vi "Mode Scan Engine.vi"() -> ()   [LabVIEW 2014]
uses:
  Controls/Standard Action.ctl
  DM_Single_V2/Controls/Standard_Counter_Action.ctl
  <vilib>/Analysis/6fits.llb/Curve Fitting Criteria.ctl
  <vilib>/Analysis/baseanly.llb/Mean (DBL).vi
  <vilib>/Analysis/NI_AALBase.lvlib
  <vilib>/Analysis/NI_AALPro.lvlib
  <vilib>/gmath/NI_Gmath.lvlib
panel:
  in  "Initial Guess":T1={"Amp"=25.0, "Center"=0.0, "Sigma"=1.0, "Offset"=0.0}
  in  "Manual Initial Guess":bool=TRUE
  in  "Upper Limit":dbl=100.0
  in  "Lower Limit":dbl=20.0
  out "Metric":cluster{dbl[], dbl[]}[](graph)
  out "Image":sgl[][](graph)
  in  "Step Size":dbl=0.5
  in  "Number of Steps":u16=9
  in  "Get Image":bool
  in  "Scan Next Mode":bool
  in  "Metric":u16(ring) items=["Max Intensity", "No Zero Mean", "Threshold Mean"]
  in  "Fit Type":u16(ring) items=["Guassian", "Quadratic"]
  in  "Mode":i32(ring) items=["1", "1"]
  in  "Apply":bool
  in  "Fit Data":bool
  in  "Scan Mode":bool
  in  "Exit":bool
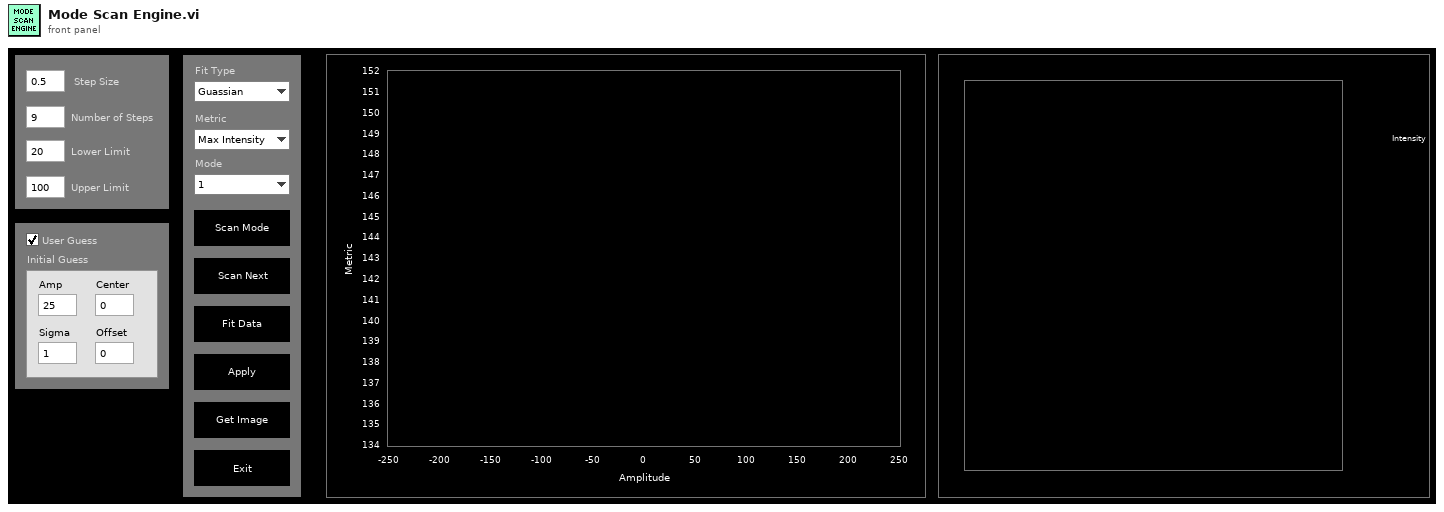
[diagram p1: front panel]
types:
  T1 = cluster{"Amp":dbl, "Center":dbl, "Sigma":dbl, "Offset":dbl}
  T2 = typedef "Standard Action.ctl" = enum16{"Read", "Write"}
  T3 = typedef "MirrorModes_DUAL.ctl" = cluster{"Mode":string, "Amplitude":dbl}[][]
  T4 = typedef "Standard_Counter_Action.ctl" = enum16{"Initialize", "Update Count", "Get Count"}
  T5 = cluster{"amp min":dbl, "amp max":dbl, "center min":dbl, "center max":dbl, "deviation min":dbl, "deviation max":dbl, "offset min":dbl, "offset max":dbl}
  T6 = enum16{"Linear", "Polynomial", "Exponential", "Power"}
  T7 = cluster{"Amplitude Out":dbl[], "Metric Out":dbl[]}
  T8 = cluster{"Amp":dbl, "Numeric":dbl, "Sigma":dbl, "Offset":dbl}
  T9 = typedef "NI_AALPro.lvlib/Curve Fitting Criteria.ctl" = u16
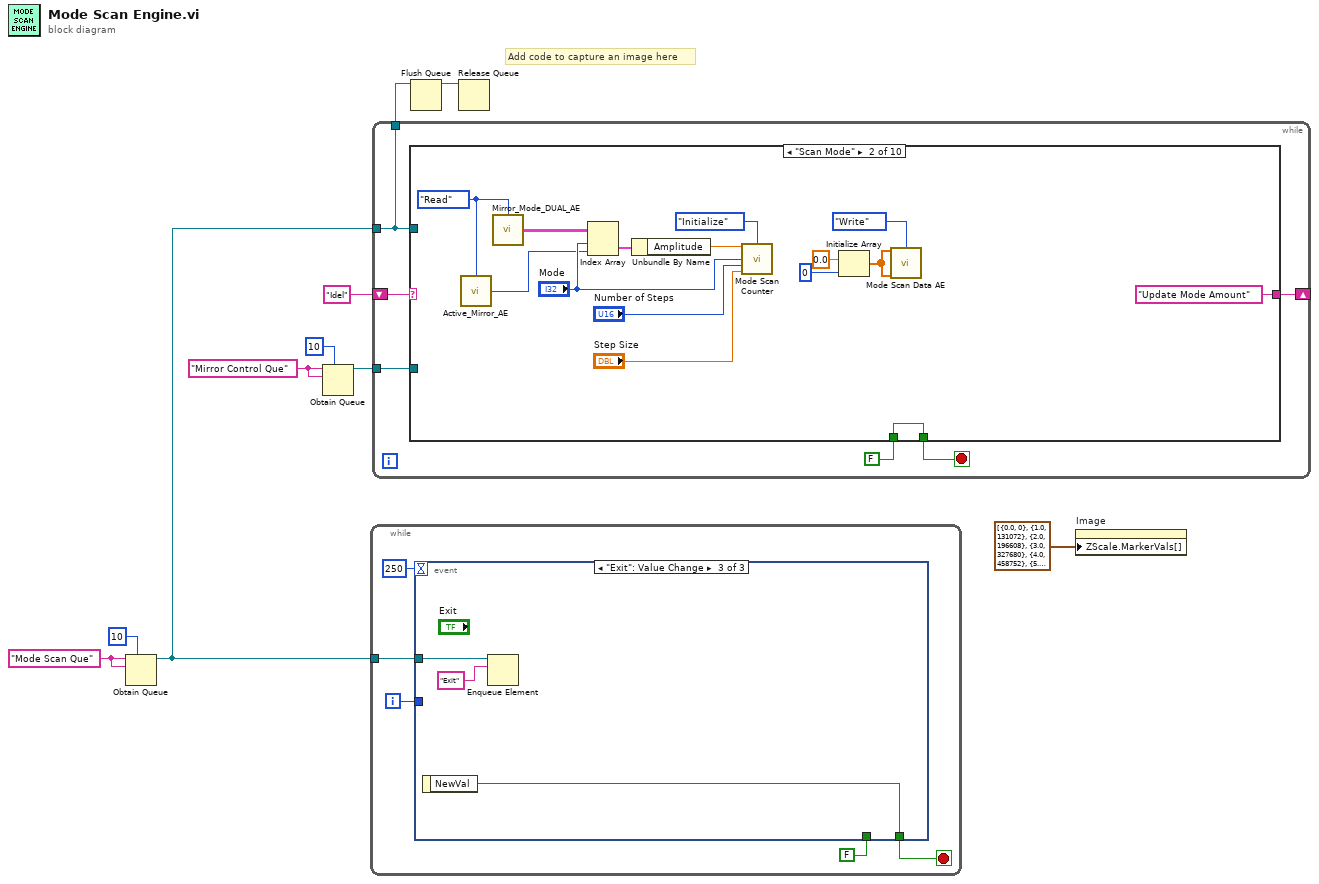
[diagram p0: block diagram]
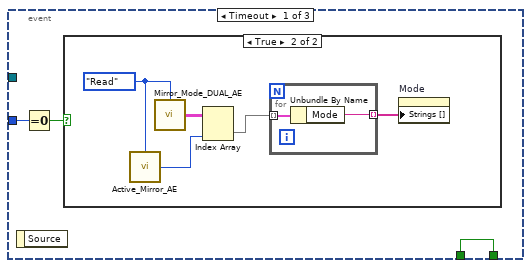
[diagram p2: hidden frame]
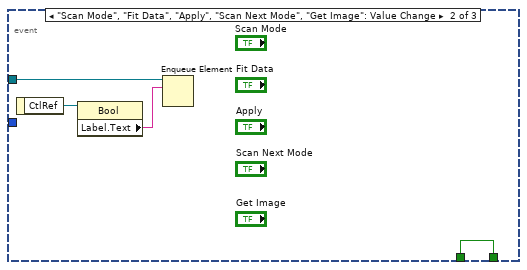
[diagram p4: hidden frame]
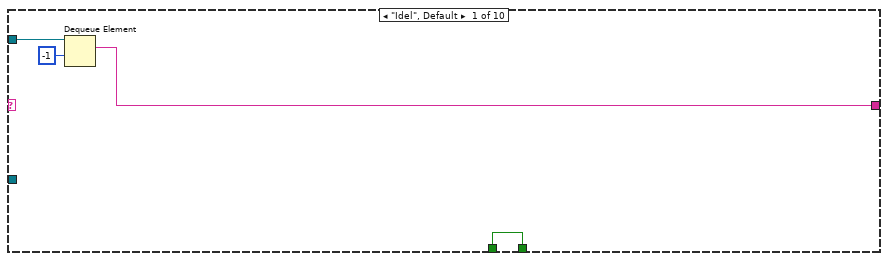
[diagram p5: hidden frame]
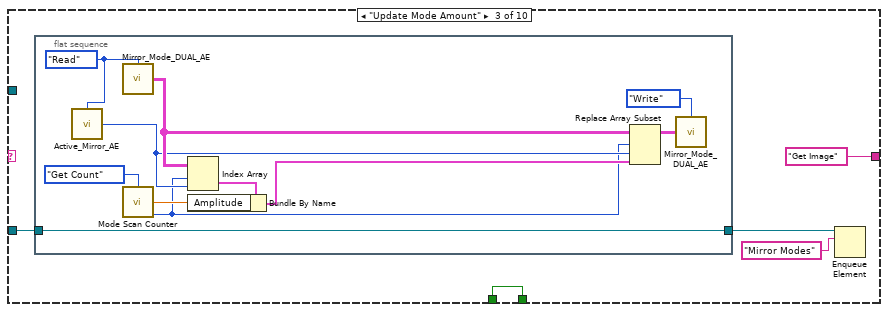
[diagram p6: hidden frame]
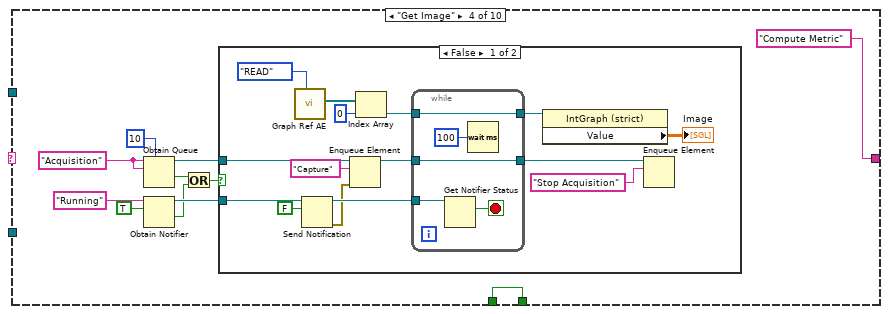
[diagram p7: hidden frame]
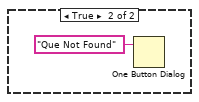
[diagram p8: hidden frame]
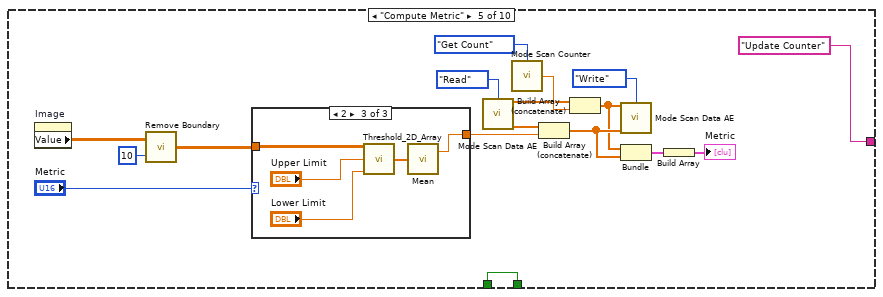
[diagram p9: hidden frame]
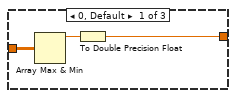
[diagram p10: hidden frame]
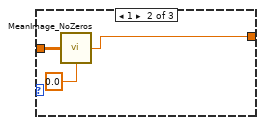
[diagram p11: hidden frame]
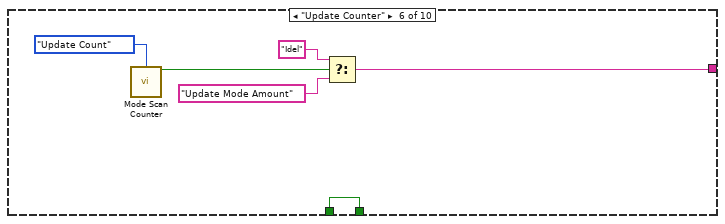
[diagram p12: hidden frame]
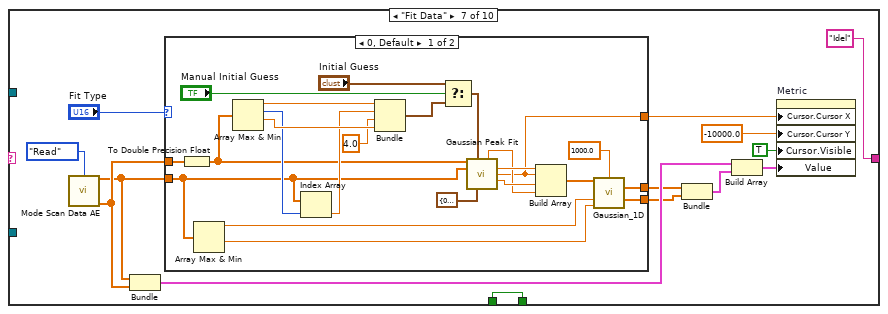
[diagram p13: hidden frame]
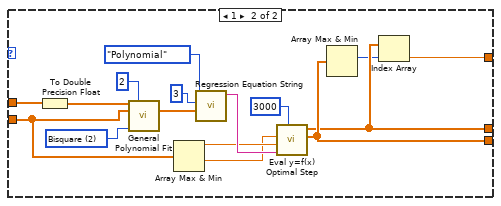
[diagram p14: hidden frame]
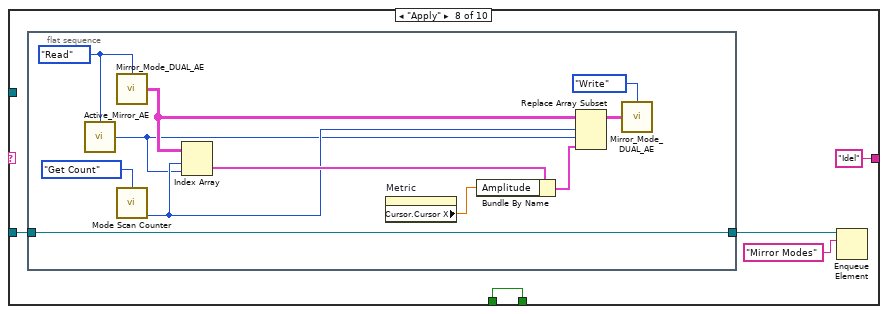
[diagram p15: hidden frame]
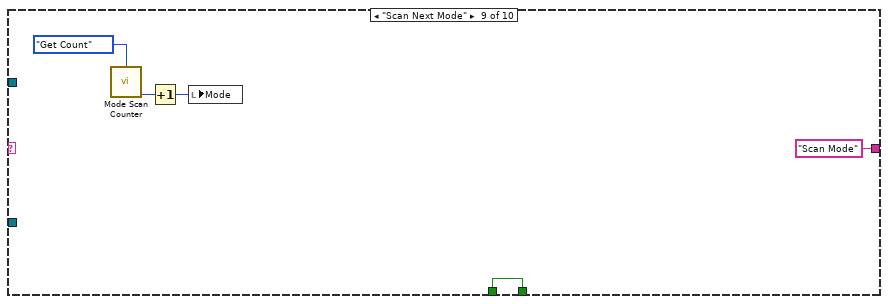
[diagram p16: hidden frame]
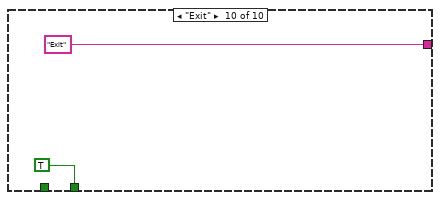
[diagram p17: hidden frame]
diagram:
  w4 = "Mirror Control Que" ("name (unnamed)")
  w9 = "Mode Scan Que" ("name (unnamed)")
  # "Add code to capture an image here"
  n1 = Obtain Queue(max queue size (-1, unlimited)=10, name (unnamed)=w9, element data type=w9) -> (queue out=w7:refnum<queue>)  [unwired: 2 in, 2 out]
  n2 = Obtain Queue(max queue size (-1, unlimited)=10, name (unnamed)=w4, element data type=w4) -> (queue out=w2:refnum<queue>)  [unwired: 2 in, 2 out]
  n3 = while {
    tunnel: w7 -> [w15]
    i -> [w12]
    stop <- w14 stop-if-true
    n4 = event shown="[2] \"Exit\": Value Change" {
      selector: _ -> [_ _ _]
      dyn-events: _ -> [_ _ _]
      timeout: 250 -> [_ _ _]
      tunnel: w15 -> [_ w28 w32]
      tunnel: [w18 w26 w30] -> w14
      tunnel: FALSE -> [w18 w26 _]
      tunnel: w12 -> [w17 _ _]
      event Timeout {
        n5 = event-data() -> ()  [unwired: 1 in, 1 out]
        n6 = Equal To 0?(x=w17) -> (x = 0?=w16:bool)
        n7 = case shown="True" w16 {
          frame False {
          }
          frame True {
            w22 = Standard_Action."Read" ("Action")
            n8 = call "Active_Mirror_AE.vi"("Action"=w22) -> ("Active Mirror"=w19:i32)  [unwired: 14 in]
            n9 = call "Mirror_Mode_DUAL_AE.vi"("Action"=w22) -> ("Mirror Modes Out"=w21:T3)  [unwired: 14 in]
            n10 = Index Array(array=w21, index (col)=w19) -> (element=w20:cluster{"Mode":string, "Amplitude":dbl}[])  [unwired: 1 in]
            n11 = for {
              tunnel: w20 -> [w25] mode=indexing
              tunnel: [w24] -> w23 mode=indexing
              n12 = Unbundle By Name(w25) -> ("Mode"=w24:string)
            }
            n13 = property on="Mode" class="Ring (strict)"("Strings []"=w23) -> ()  [unwired: 2 in, 2 out]
          }
        }
      }
      event "Scan Mode", "Fit Data", "Apply", "Scan Next Mode", "Get Image": Value Change {
        n14 = event-data() -> ("CtlRef"=w27:refnum<vi>)  [unwired: 1 in]
        n15 = property class="Bool"(reference=w27) -> ("Label.Text"=w29:string)  [unwired: 1 in, 2 out]
        n16 = Enqueue Element(queue=w28, element=w29) -> ()  [unwired: 2 in, 3 out]
      }
      event "Exit": Value Change {
        n17 = event-data() -> ("NewVal"=w30:bool)  [unwired: 1 in]
        n18 = Enqueue Element(queue=w32, element="Exit") -> ()  [unwired: 2 in, 3 out]
      }
    }
  }
  n19 = while {
    shift-right: [w35] -> _
    shift-left: "Idel" -> [w38]
    tunnel: w7 -> [w34]
    tunnel: [w34] -> w6
    tunnel: w2 -> [w33]
    stop <- w37 stop-if-true
    n20 = case shown="\"Scan Mode\"" w38 {
      tunnel: [w42 w57 w62 w84 w121 w139 w153 w197 w213 TRUE] -> w37
      tunnel: FALSE -> [w42 w57 w62 w84 w121 w139 w153 w197 w213 _]
      tunnel: w34 -> [w40 _ _ _ _ _ _ _ _ _]
      tunnel: [w39 "Update Mode Amount" ("name (unnamed)") "Get Image" ("name (unnamed)") "Compute Metric" ("name (unnamed)") "Update Counter" ("name (unnamed)") w136 "Idel" ("name (unnamed)") "Idel" ("name (unnamed)") "Scan Mode" ("name (unnamed)") "Exit" ("name (unnamed)")] -> w35
      tunnel: w33 -> [_ _ w61 _ _ _ _ w195 _ _]
      frame "Idel", Default {
        n21 = Dequeue Element(queue=w40, timeout in ms (-1)=-1) -> (element=w39:string)  [unwired: 1 in, 3 out]
      }
      frame "Scan Mode" {
        w45 = Standard_Action."Read" ("Action")
        n22 = call "Active_Mirror_AE.vi"("Action"=w45) -> ("Active Mirror"=w43:i32)  [unwired: 14 in]
        n23 = call "Mirror_Mode_DUAL_AE.vi"("Action"=w45) -> ("Mirror Modes Out"=w52:T3)  [unwired: 14 in]
        n24 = Index Array(array=w52, index (row)="Mode", index (col)=w43) -> (element=w53:cluster{"Mode":string, "Amplitude":dbl})
        n25 = Unbundle By Name(w53) -> ("Amplitude"=w54:dbl)
        n26 = call "Mode Scan Counter.vi"("Center Value"=w54, "Action"=Standard_Counter_Action."Initialize", "Mode"="Mode", "Number of Steps"="Number of Steps", "Step Size"="Step Size") -> ()  [unwired: 8 in, 3 out]
        n27 = Initialize Array(0.0 ("element"), 0 ("dimension size")) -> (w46:dbl[])
        n28 = call "Mode Scan Data AE.vi"("Amplitude"=w46, "Action"=Standard_Action."Write", "Metric"=w46) -> ()  [unwired: 11 in, 2 out]
      }
      frame "Update Mode Amount" {
        n29 = flat-sequence {
          tunnel: w61 -> [w66]
          tunnel: [w66] -> w59
          frame #0 {
            w65 = Standard_Action."Read" ("Action")
            n30 = call "Active_Mirror_AE.vi"("Action"=w65) -> ("Active Mirror"=w64:i32)  [unwired: 14 in]
            n31 = call "Mirror_Mode_DUAL_AE.vi"("Action"=w65) -> ("Mirror Modes Out"=w68:T3)  [unwired: 14 in]
            n32 = call "Mode Scan Counter.vi"("Action"=Standard_Counter_Action."Get Count") -> ("Output"=w72:dbl, "Current Mode"=w63:i32)  [unwired: 12 in, 1 out]
            n33 = Index Array(array=w68, index (row)=w63, index (col)=w64) -> (element=w71:cluster{"Mode":string, "Amplitude":dbl})
            n34 = Bundle By Name(cluster=w71, "Amplitude"=w72) -> (w73:cluster{"Mode":string, "Amplitude":dbl})
            n35 = Replace Array Subset(array=w68, new element=w73, index (row)=w63, index (col)=w64) -> (w70:T3)
            n36 = call "Mirror_Mode_DUAL_AE.vi"("Action"=Standard_Action."Write", "Mirror Modes In"=w70) -> ()  [unwired: 13 in, 1 out]
          }
        }
        n37 = Enqueue Element(queue=w59, element="Mirror Modes" ("name (unnamed)")) -> ()  [unwired: 2 in, 3 out]
      }
      frame "Get Image" {
        w79 = "Acquisition" ("name (unnamed)")
        n38 = Obtain Queue(max queue size (-1, unlimited)=10, name (unnamed)=w79, element data type=w79) -> (queue out=w82:refnum<queue>, created new?=w76:bool)  [unwired: 2 in, 1 out]
        n39 = Obtain Notifier(name (unnamed)="Running", notification data type=TRUE) -> (notifier out=w81:refnum<notifier>, created new?=w75:bool)  [unwired: 2 in, 1 out]
        n40 = Or(x=w76, y=w75) -> (x .or. y?=w74:bool)
        n41 = case shown="False" w74 {
          tunnel: w82 -> [w88 _]
          tunnel: w81 -> [w86 _]
          frame False {
            n42 = call "Graph Ref AE.vi"("Action"=enum16{"READ", "WRITE"}."READ") -> ("Graph Ref Out"=w96:refnum<vi>[])  [unwired: 10 in]
            n43 = Send Notification(notification=FALSE, notifier=w86) -> (notifier out=w91:refnum<notifier>, error out=w90:errorcluster)  [unwired: 1 in]
            n44 = Enqueue Element(queue=w88, element="Capture", error in (no error)=w90) -> (queue out=w92:refnum<queue>)  [unwired: 1 in, 2 out]
            n45 = Index Array(array=w96, index=0) -> (element=w98:refnum<vi>)
            n46 = while {
              tunnel: w91 -> [w104]
              tunnel: [w102] -> w93
              tunnel: w92 -> [w102]
              tunnel: [w101] -> w99
              tunnel: w98 -> [w101]
              stop <- w103 stop-if-true
              n47 = Get Notifier Status(notifier=w104) -> (current notification=w103:bool)  [unwired: 1 in, 4 out]
              n48 = Wait (ms)(milliseconds to wait=u32 100) -> ()  [unwired: 1 out]
            }
            n49 = property class="IntGraph (strict)"(reference=w99) -> ("Value"=→"Image":sgl[][])  [unwired: 1 in, 2 out]
            n50 = Enqueue Element(queue=w93, element="Stop Acquisition" ("f")) -> ()  [unwired: 2 in, 3 out]
          }
          frame True {
            n51 = One Button Dialog(message="Que Not Found") -> ()  [unwired: 1 in, 1 out]
          }
        }
      }
      frame "Compute Metric" {
        n52 = property on="Image" class="IntGraph (strict)"() -> ("Value"=w108:sgl[][])  [unwired: 2 in, 2 out]
        n53 = call "Remove Boundary.vi"("deleted pixel number"=10, "input"=w108) -> ("output"=w107:dbl[][])
        n54 = case shown="2" "Metric" {
          tunnel: w107 -> [w125 w128 w133]
          tunnel: [w123 w127 w131] -> w115
          frame 0, Default {
            n55 = Array Max & Min(array=w125) -> (max value=w124:dbl)  [unwired: 3 out]
            n56 = To Double Precision Float(number=w124) -> (double precision float=w123:dbl)
          }
          frame 1 {
            n57 = call "MeanImage_NoZeros.vi"("Image IN"=w128, "STDev Factor"=0.0) -> ("No Zero Mean"=w127:dbl)  [unwired: 13 in]
          }
          frame 2 {
            n58 = call "Threshold_2D_Array.vi"("2D Array IN"=w133, "Upper Limit"="Upper Limit", "Lower Limit"="Lower Limit") -> ("Threshold Array Out"=w132:dbl[])  [unwired: 12 in]
            n59 = call-poly <vilib>:"Mean.vi"("X"=w132) -> ("mean"=w131:dbl)  [unwired: 1 out]
          }
        }
        n60 = call "Mode Scan Data AE.vi"("Action"=Standard_Action."Read") -> ("Amplitude Out"=w112:dbl[], "Metric Out"=w113:dbl[])  [unwired: 13 in]
        n61 = call "Mode Scan Counter.vi"("Action"=Standard_Counter_Action."Get Count") -> ("Output"=w114:dbl)  [unwired: 12 in, 2 out]
        n62 = Build Array (concatenate)(w113, w115) -> (w118:dbl[])
        n63 = Build Array (concatenate)(w112, w114) -> (w117:dbl[])
        n64 = call "Mode Scan Data AE.vi"("Amplitude"=w117, "Action"=Standard_Action."Write", "Metric"=w118) -> ()  [unwired: 11 in, 2 out]
        n65 = Bundle(w117, w118) -> (w119:cluster{dbl[], dbl[]})  [unwired: 1 in]
        n66 = Build Array(w119) -> (→"Metric":cluster{dbl[], dbl[]}[])
      }
      frame "Update Counter" {
        n67 = call "Mode Scan Counter.vi"("Action"=Standard_Counter_Action."Update Count") -> ("Scan Done?"=w134:bool)  [unwired: 12 in, 2 out]
        n68 = Select(t="Idel", s=w134, f="Update Mode Amount") -> (s? t:f=w136:string)
      }
      frame "Fit Data" {
        n69 = call "Mode Scan Data AE.vi"("Action"=Standard_Action."Read") -> ("Amplitude Out"=w148:dbl[], "Metric Out"=w149:dbl[])  [unwired: 13 in]
        n70 = Bundle("Amplitude Out"=w148, "Metric Out"=w149) -> (w147:T7)  [unwired: 1 in]
        n71 = case shown="0, Default" "Fit Type" {
          tunnel: w148 -> [w169 w182]
          tunnel: w149 -> [w176 w181]
          tunnel: [w157 w178] -> w142
          tunnel: [w156 w179] -> w145
          tunnel: [w155 w180] -> w144
          frame 0, Default {
            n72 = To Double Precision Float(number=w176) -> (double precision float=w170:dbl[])
            n73 = Array Max & Min(array=w169) -> (max value=w158:dbl, min value=w159:dbl)  [unwired: 2 out]
            n74 = Array Max & Min(array=w170) -> (max value=w175:dbl, max index (indices)=w172:i32, min value=w174:dbl)  [unwired: 1 out]
            n75 = Index Array(array=w169, index=w172) -> (element=w171:dbl)
            n76 = Bundle(w175, "Numeric"=w171, 4.0, w174) -> (w168:cluster{dbl, "Numeric":dbl, dbl, dbl})  [unwired: 1 in]
            n77 = Select(t="Initial Guess", s="Manual Initial Guess", f=w168) -> (s? t:f=w167:T8)
            n78 = call <vilib>:"Gaussian Peak Fit.vi"("Y"=w170, "initial guess"=w167, "X"=w169, "parameter bounds"=T5 {"amp min"=0.0, "amp max"=100000.0, "center min"=-100.0, "center max"=100.0, "deviation min"=0.0, "deviation max"=1000.0, "offset min"=0.0, "offset max"=1000.0}) -> ("offset"=w162:dbl, "amplitude"=w164:dbl, "center"=w157:dbl, "standard deviation"=w163:dbl)  [unwired: 5 in, 3 out]
            n79 = Build Array(w164, w157, w163, w162) -> (w161:dbl[])
            n80 = call "Gaussian_1D.vi"("Parameters In"=w161, "Number of Points"=1000.0, "Max X Value"=w158, "Min X Value"=w159) -> ("X Values"=w156:dbl[], "Y Values"=w155:dbl[])  [unwired: 10 in]
          }
          frame 1 {
            w191 = T9 2 items=["Least Square", "Least Absolute Residual", "Bisquare"] ("method")
            n81 = To Double Precision Float(number=w181) -> (double precision float=w192:dbl[])
            n82 = call <vilib>:"General Polynomial Fit.vi"("Y"=w192, "polynomial order"=2, "X"=w182, "method"=w191) -> ("Polynomial Coefficients"=w188:dbl[])  [unwired: 8 in, 3 out]
            n83 = Array Max & Min(array=w182) -> (max value=w184:dbl, min value=w183:dbl)  [unwired: 2 out]
            n84 = call "Regression Equation String.vi"("coefficients"=w188, "precision"=3, "fit type"=T6."Polynomial") -> ("Formula"=w186:string)  [unwired: 8 in]
            n85 = call <vilib>:"Eval y=f(x) Optimal Step.vi"("number of points"=u32 3000, "formula"=w186, "end"=w184, "start"=w183) -> ("Y Values"=w180:dbl[], "X Values"=w179:dbl[])  [unwired: 1 in, 2 out]
            n86 = Array Max & Min(array=w180) -> (max index (indices)=w177:i32)  [unwired: 3 out]
            n87 = Index Array(array=w179, index=w177) -> (element=w178:dbl)
          }
        }
        n88 = Bundle("X Values"=w145, "Y Values"=w144) -> (w143:cluster{"X Values":dbl[], "Y Values":dbl[]})  [unwired: 1 in]
        n89 = Build Array(w147, w143) -> (w146:cluster{"X Values":dbl[], "Y Values":dbl[]}[])
        n90 = property on="Metric" class="XYGraph (strict)"("Cursor.Cursor X"=w142, "Cursor.Cursor Y"=-10000.0 ("Cursor.Cursor Position:Cursor X"), "Cursor.Visible"=TRUE, "Value"=w146) -> ()  [unwired: 2 in, 2 out]
      }
      frame "Apply" {
        n91 = flat-sequence {
          tunnel: [w202] -> w193
          tunnel: w195 -> [w202]
          frame #0 {
            w200 = Standard_Action."Read" ("Action")
            n92 = call "Active_Mirror_AE.vi"("Action"=w200) -> ("Active Mirror"=w198:i32)  [unwired: 14 in]
            n93 = call "Mirror_Mode_DUAL_AE.vi"("Action"=w200) -> ("Mirror Modes Out"=w204:T3)  [unwired: 14 in]
            n94 = call "Mode Scan Counter.vi"("Action"=Standard_Counter_Action."Get Count") -> ("Current Mode"=w199:i32)  [unwired: 12 in, 2 out]
            n95 = Index Array(array=w204, index (row)=w199, index (col)=w198) -> (element=w207:cluster{"Mode":string, "Amplitude":dbl})
            n96 = property on="Metric" class="XYGraph (strict)"() -> ("Cursor.Cursor X"=w201:dbl)  [unwired: 2 in, 2 out]
            n97 = Bundle By Name(cluster=w207, "Amplitude"=w201) -> (w208:cluster{"Mode":string, "Amplitude":dbl})
            n98 = Replace Array Subset(array=w204, new element=w208, index (row)=w199, index (col)=w198) -> (w206:T3)
            n99 = call "Mirror_Mode_DUAL_AE.vi"("Action"=Standard_Action."Write", "Mirror Modes In"=w206) -> ()  [unwired: 13 in, 1 out]
          }
        }
        n100 = Enqueue Element(queue=w193, element="Mirror Modes" ("name (unnamed)")) -> ()  [unwired: 2 in, 3 out]
      }
      frame "Scan Next Mode" {
        n101 = call "Mode Scan Counter.vi"("Action"=Standard_Counter_Action."Get Count") -> ("Current Mode"=w210:i32)  [unwired: 12 in, 2 out]
        n102 = Increment(x=w210) -> (x+1=w211:i32)
        n103 = local write "Mode"(w211) -> ()
      }
      frame "Exit" {
      }
    }
  }
  n104 = Flush Queue(queue=w6) -> (queue out=w5:refnum<queue>)  [unwired: 1 in, 2 out]
  n105 = Release Queue(queue=w5) -> ()  [unwired: 2 in, 3 out]
  n106 = property on="Image" class="IntGraph (strict)"("ZScale.MarkerVals[]"=cluster{dbl, u32}[] [{0.0, 0}, {1.0, 131072}, {2.0, 196608}, {3.0, 327680}, {4.0, 458752}, {5.0, 589824}, {6.0, 720896}, {7.0, 851971}, {8.0, 983043}, {9.0, 1114115}, {10.0, 1245187}, {11.0, 1376259}, {12.0, 1507331}, {13.0, 1638403}, {14.0, 1769475}, {15.0, 1769479}, {16.0, 2031623}, {17.0, 2162695}, {18.0, 2293767}, {19.0, 2424839}, {20.0, 2555911}, {21.0, 2686983}, {22.0, 2818055}, {23.0, 2949127}, {24.0, 3080203}, {25.0, 3211275}, {26.0, 3342347}, {27.0, 3473419}, {28.0, 3604491}, {29.0, 3735563}, {30.0, 3866635}, {31.0, 3867403}, {32.0, 4129547}, {33.0, 4260619}, {34.0, 4391691}, {35.0, 4522763}, {36.0, 4653839}, {37.0, 4784911}, {38.0, 4915983}, {39.0, 5178127}, {40.0, 5309199}, {41.0, 5440271}, {42.0, 5571343}, {43.0, 5702415}, {44.0, 5703439}, {45.0, 5965583}, {46.0, 6096655}, {47.0, 6227727}, {48.0, 6358799}, {49.0, 6489871}, {50.0, 6620943}, {51.0, 6752015}, {52.0, 6883087}, {53.0, 7015183}, {54.0, 7146255}, {55.0, 7277327}, {56.0, 7408399}, {57.0, 7539471}, {58.0, 7670543}, {59.0, 7801615}, {60.0, 8063759}, {61.0, 8194831}, {62.0, 8326927}, {63.0, 8457999}, {64.0, 8589075}, {65.0, 8720147}, {66.0, 8851219}, {67.0, 8982291}, {68.0, 9113363}, {69.0, 9114387}, {70.0, 9376531}, {71.0, 9507603}, {72.0, 9638675}, {73.0, 9769747}, {74.0, 9901843}, {75.0, 10032915}, {76.0, 10163987}, {77.0, 10229523}, {78.0, 10295059}, {79.0, 10427155}, {80.0, 10558227}, {81.0, 10689299}, {82.0, 10820371}, {83.0, 10886931}, {84.0, 10952467}, {85.0, 11083539}, {86.0, 11214611}, {87.0, 11215635}, {88.0, 11477779}, {89.0, 11543315}, {90.0, 11608851}, {91.0, 11740947}, {92.0, 11806483}, {93.0, 11872019}, {94.0, 12004115}, {95.0, 12135187}, {96.0, 12266259}, {97.0, 12267283}, {98.0, 12398355}, {99.0, 12529427}, {100.0, 12530451}, {101.0, 12595987}, {102.0, 12530451}, {103.0, 12793619}, {104.0, 12794131}, {105.0, 12794643}, {106.0, 13056787}, {107.0, 13057299}, {108.0, 13057811}, {109.0, 13188883}, {110.0, 13320979}, {111.0, 13386515}, {112.0, 13452563}, {113.0, 13584147}, {114.0, 13584659}, {115.0, 13585171}, {116.0, 13585683}, {117.0, 13717267}, {118.0, 13848339}, {119.0, 13849363}, {120.0, 13849875}, {121.0, 13850387}, {122.0, 13981459}, {123.0, 14113555}, {124.0, 14114067}, {125.0, 14114579}, {126.0, 14115091}, {127.0, 14246675}, {128.0, 14377747}, {129.0, 14378771}, {130.0, 14379283}, {131.0, 14379539}, {132.0, 14379795}, {133.0, 14380819}, {134.0, 14511891}, {135.0, 14643987}, {136.0, 14644503}, {137.0, 14645015}, {138.0, 14645527}, {139.0, 14646039}, {140.0, 14646551}, {141.0, 14778135}, {142.0, 14909207}, {143.0, 14910231}, {144.0, 14910747}, {145.0, 14911259}, {146.0, 14911771}, {147.0, 14912283}, {148.0, 14912797}, {149.0, 15044383}, {150.0, 15175455}, {151.0, 15175967}, {152.0, 15176479}, {153.0, 15176991}, {154.0, 15177507}, {155.0, 15178019}, {156.0, 15178531}, {157.0, 15310115}, {158.0, 15441701}, {159.0, 15441959}, {160.0, 15442215}, {161.0, 15442727}, {162.0, 15443243}, {163.0, 15443755}, {164.0, 15444269}, {165.0, 15444783}, {166.0, 15444783}, {167.0, 15576367}, {168.0, 15707953}, {169.0, 15708467}, {170.0, 15708979}, {171.0, 15708981}, {172.0, 15708983}, {173.0, 15710011}, {174.0, 15710523}, {175.0, 15711037}, {176.0, 15711039}, {177.0, 15711553}, {178.0, 15843139}, {179.0, 15974213}, {180.0, 15974215}, {181.0, 15974217}, {182.0, 15974219}, {183.0, 15975755}, {184.0, 15976271}, {185.0, 15976785}, {186.0, 15977299}, {187.0, 15977301}, {188.0, 15977815}, {189.0, 15978327}, {190.0, 15978331}, {191.0, 16109917}, {192.0, 16241503}, {193.0, 16241505}, {194.0, 16242019}, {195.0, 16242535}, {196.0, 16242537}, {197.0, 16242539}, {198.0, 16243563}, {199.0, 16243567}, {200.0, 16244081}, {201.0, 16244595}, {202.0, 16244599}, {203.0, 16244601}, {204.0, 16244603}, {205.0, 16245627}, {206.0, 16245631}, {207.0, 16245633}, {208.0, 16246147}, {209.0, 16246663}, {210.0, 16377735}, {211.0, 16508811}, {212.0, 16508815}, {213.0, 16509839}, {214.0, 16509843}, {215.0, 16509845}, {216.0, 16509847}, {217.0, 16510361}, {218.0, 16510875}, {219.0, 16510879}, {220.0, 16510881}, {221.0, 16510883}, {222.0, 16511399}, {223.0, 16511911}, {224.0, 16511915}, {225.0, 16511917}, {226.0, 16511919}, {227.0, 16511923}, {228.0, 16512437}, {229.0, 16512951}, {230.0, 16512955}, {231.0, 16512957}, {232.0, 16512959}, {233.0, 16512961}, {234.0, 16512963}, {235.0, 16512967}, {236.0, 16513481}, {237.0, 16513995}, {238.0, 16513999}, {239.0, 16514001}, {240.0, 16514003}, {241.0, 16514005}, {242.0, 16514007}, {243.0, 16514011}, {244.0, 16514013}, {245.0, 16514015}, {246.0, 16514019}, {247.0, 16514021}, {248.0, 16514023}, {249.0, 16514027}, {250.0, 16514029}, {251.0, 16514031}, {252.0, 16514035}, {253.0, 16514037}, {254.0, 16514039}, {255.0, 16514043}] ("Z Scale.Marker Values[]")) -> ()  [unwired: 2 in, 2 out]
